vi "Vertex.vi"(8 "Index":i32, 10 "Point2D":T1, 11 "DocIn":refnum<k20>) -> (2 "Vertex":refnum<k20>, 3 "DocOut":refnum<k20>)   [LabVIEW 2014]
uses:
  TypeDefs/Point2DwSlope.ctl
  <resource>/objmgr/DOMUserDefRef.rc
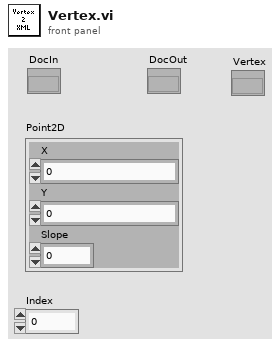
[diagram p1: front panel]
types:
  T1 = typedef "Point2DwSlope.ctl" = cluster{"X":sgl, "Y":sgl, "Slope":dbl}
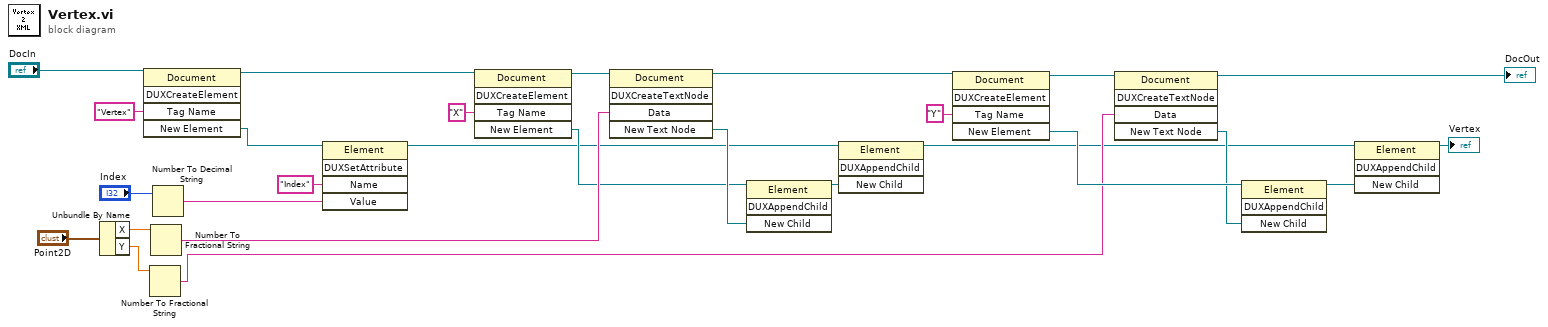
[diagram p0: block diagram]
diagram:
  n1 = Unbundle By Name("Point2D") -> ("X"=w25:sgl, "Y"=w24:sgl)
  n2 = invoke class="Document" method="DUXCreateElement"(reference="DocIn", "Tag Name"="Vertex") -> (reference out=w11:refnum<k20>, "New Element"=w12:refnum<k20>)  [unwired: 3 in, 3 out]
  n3 = Number To Fractional String(number=w24) -> (F-format string=w13:string)  [unwired: 3 in]
  n4 = Number To Fractional String(number=w25) -> (F-format string=w21:string)  [unwired: 3 in]
  n5 = Number To Decimal String(number="Index") -> (decimal integer string=w9:string)  [unwired: 1 in]
  n6 = invoke class="Element" method="DUXSetAttribute"(reference=w12, "Name"="Index", "Value"=w9) -> (reference out=w7:refnum<k20>)  [unwired: 2 in, 4 out]
  n7 = invoke class="Document" method="DUXCreateElement"(reference=w11, "Tag Name"="X") -> (reference out=w22:refnum<k20>, "New Element"=w19:refnum<k20>)  [unwired: 3 in, 3 out]
  n8 = invoke class="Document" method="DUXCreateTextNode"(reference=w22, "Data"=w21) -> (reference out=w14:refnum<k20>, "New Text Node"=w20:refnum<k20>)  [unwired: 3 in, 3 out]
  n9 = invoke class="Element" method="DUXAppendChild"(reference=w19, "New Child"=w20) -> (reference out=w4:refnum<k20>)  [unwired: 2 in, 3 out]
  n10 = invoke class="Element" method="DUXAppendChild"(reference=w7, "New Child"=w4) -> (reference out=w6:refnum<k20>)  [unwired: 2 in, 3 out]
  n11 = invoke class="Document" method="DUXCreateElement"(reference=w14, "Tag Name"="Y") -> (reference out=w16:refnum<k20>, "New Element"=w18:refnum<k20>)  [unwired: 3 in, 3 out]
  n12 = invoke class="Document" method="DUXCreateTextNode"(reference=w16, "Data"=w13) -> (reference out=→"DocOut":refnum<k20>, "New Text Node"=w17:refnum<k20>)  [unwired: 3 in, 3 out]
  n13 = invoke class="Element" method="DUXAppendChild"(reference=w18, "New Child"=w17) -> (reference out=w5:refnum<k20>)  [unwired: 2 in, 3 out]
  n14 = invoke class="Element" method="DUXAppendChild"(reference=w6, "New Child"=w5) -> (reference out=→"Vertex":refnum<k20>)  [unwired: 2 in, 3 out]
